vi "Delivery Notifier Handler.vi"(7 "Command (Store)":T1=enum."Store", 8 "error in":errorcluster, 10 "Delivery Notifier":refnum<notifier>) -> (0 "error out":errorcluster)   [LabVIEW 2016, in "Optimization Framework.lvlib" / "Optimization.lvclass"]
uses:
  Optimization.lvclass
  Delivery Notifier Handler Command.ctl
  <vilib>/ActorFramework/Time-Delayed Send Message/Time-Delay Override Options.ctl
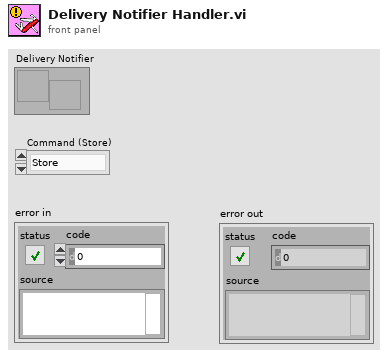
[diagram p1: front panel]
types:
  T1 = typedef "Optimization Framework.lvlib/Optimization.lvclass/Delivery Notifier Handler Command.ctl" = enum16{"Initiate", "Store", "Close All"}
  T2 = typedef "Time-Delay Override Options.ctl" = enum16{"Send next copy now", "Skip next scheduled copy", "Send next copy now and stop all further copies", "Stop all further copies"}
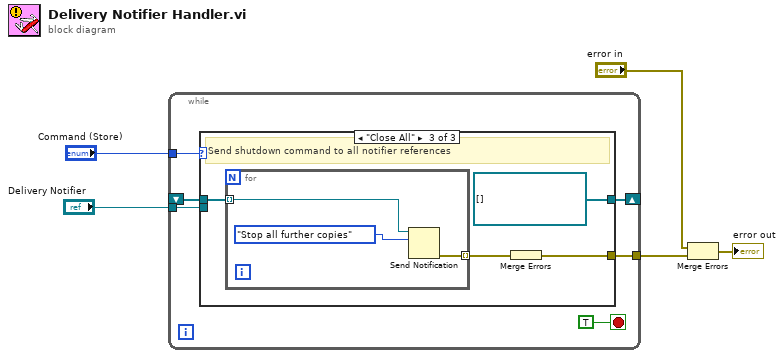
[diagram p0: block diagram]
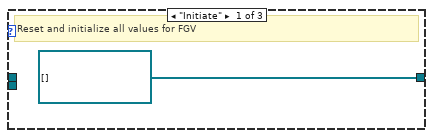
[diagram p2: hidden frame]
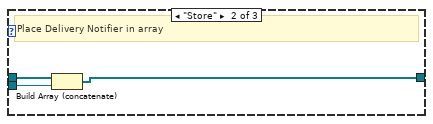
[diagram p3: hidden frame]
diagram:
  n1 = while {
    tunnel: [w10] -> w5
    tunnel: "Command (Store)" -> [w9]
    shift-right: [w8] -> _
    shift-left: _ -> [w7]
    tunnel: "Delivery Notifier" -> [w6]
    stop <- TRUE stop-if-true
    n2 = case shown="\"Close All\"" w9 {
      tunnel: [_ _ w16] -> w10
      tunnel: [w12 w13 w18] -> w8
      tunnel: w7 -> [_ w15 w19]
      tunnel: w6 -> [_ w14 _]
      frame "Initiate" {
        w12 = refnum<notifier>[] [] items=["Send next copy now", "Skip next scheduled copy", "Send next copy now and stop all further copies", "Stop all further copies"] ("Delivery Notifier")
        # "Reset and initialize all values for FGV"
      }
      frame "Store" {
        # "Place Delivery Notifier in array"
        n3 = Build Array (concatenate)(w15, w14) -> (w13:refnum<notifier>[])
      }
      frame "Close All" {
        w18 = refnum<notifier>[] [] items=["Send next copy now", "Skip next scheduled copy", "Send next copy now and stop all further copies", "Stop all further copies"] ("Delivery Notifier")
        # "Send shutdown command to all notifier references"
        n4 = for {
          tunnel: w19 -> [w22] mode=indexing
          tunnel: [w20] -> w17 mode=indexing
          n5 = Send Notification(notification=Time-Delay_Override_Options."Stop all further copies", notifier=w22) -> (error out=w20:errorcluster)  [unwired: 1 in, 1 out]
        }
        n6 = Merge Errors(w17) -> (w16:errorcluster)
      }
    }
  }
  n7 = Merge Errors("error in", w5) -> (→"error out":errorcluster)
